vi "Ouputs to Tag Bus.vi"(11 "tag bus in":T1) -> (3 "tag bus out":T1)   [LabVIEW 2015, in "PID Module 2 runtime.lvclass"]
uses:
  PID Module 2 runtime.lvclass
  <vilib>/NI/Tag Bus/table/data table.ctl
  <vilib>/NI/Tag Bus/table/data polymorphs/write one/write Double.vi
  <vilib>/NI/Tag Bus/table/data table.lvlib
panel:
  in  "Outputs index":i32[](array[numeric])
  in  "output in":dbl[](array[numeric])
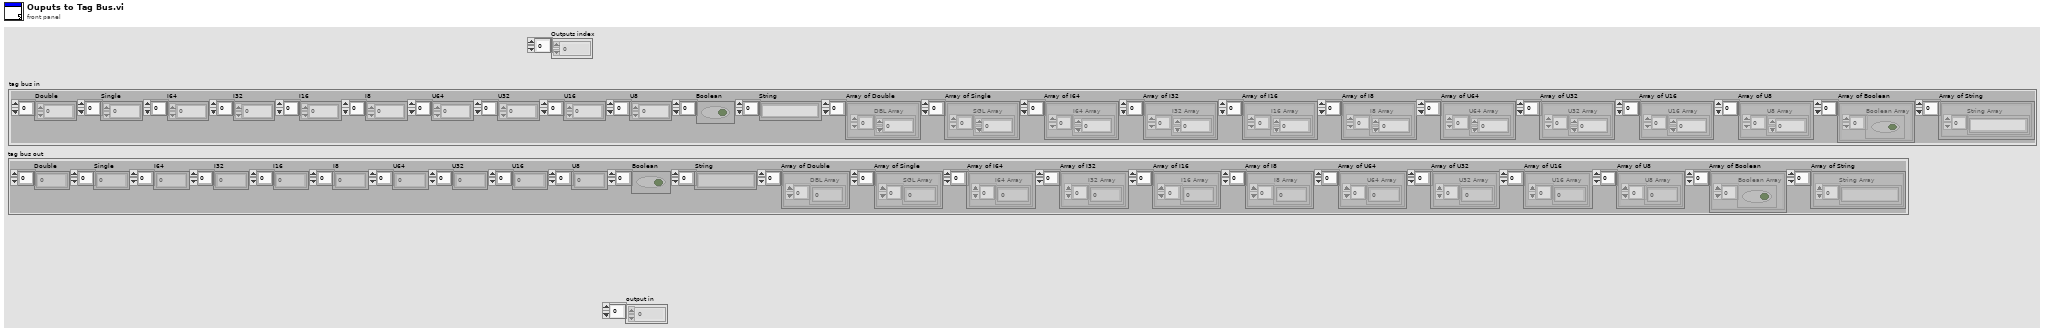
[diagram p1: front panel]
types:
  T1 = typedef "tag bus.lvlib/data table.lvlib/data table.ctl" = cluster{"Double":dbl[], "Single":sgl[], "I64":i64[], "I32":i32[], "I16":i16[], "I8":i8[], "U64":u64[], "U32":u32[], "U16":u16[], "U8":u8[], "Boolean":bool[], "String":string[], "Array of Double":cluster{"DBL Array":dbl[]}[], "Array of Single":cluster{"SGL Array":sgl[]}[], "Array of I64":cluster{"I64 Array":i64[]}[], "Array of I32":cluster{"I32 Array":i32[]}[], "Array of I16":cluster{"I16 Array":i16[]}[], "Array of I8":cluster{"I8 Array":i8[]}[], "Array of U64":cluster{"U64 Array":u64[]}[], "Array of U32":cluster{"U32 Array":u32[]}[], "Array of U16":cluster{"U16 Array":u16[]}[], "Array of U8":cluster{"U8 Array":u8[]}[], "Array of Boolean":cluster{"Boolean Array":bool[]}[], "Array of String":cluster{"String Array":string[]}[]}
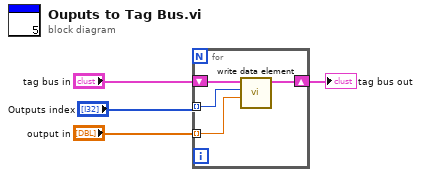
[diagram p0: block diagram]
diagram:
  n1 = for {
    shift-right: [w7] -> w3
    shift-left: "tag bus in" -> [w8]
    tunnel: "output in" -> [w6] mode=indexing
    tunnel: "Outputs index" -> [w5] mode=indexing
    n2 = call-poly <vilib>:"write data element.vi"("value"=w6, "index"=w5, "data table in"=w8) -> ("data table out"=w7:T1)  [unwired: 8 in]
  }
  "tag bus out" <- w3
